vi "运行模式解析.vi"(1 "中英文选择":enum32{"中文", "English"}(radio), 2 "输入值":u8) -> (0 "输出值":string)   [LabVIEW 2013]
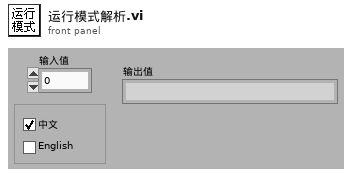
[diagram p1: front panel]
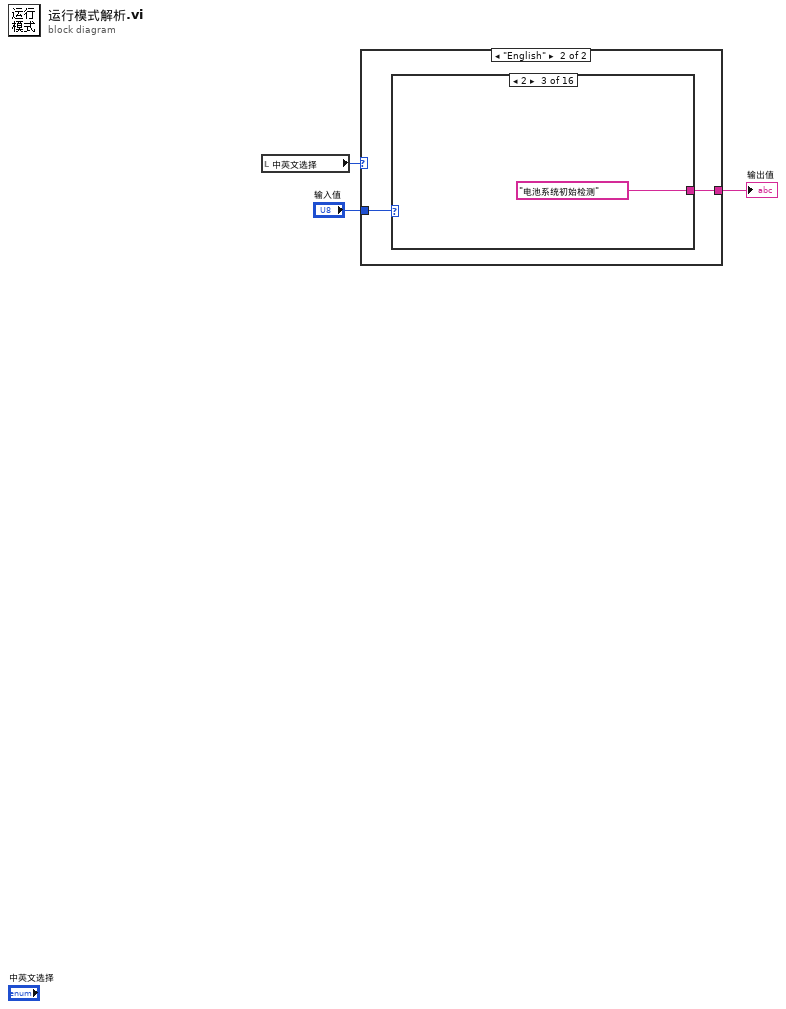
[diagram p0: block diagram]
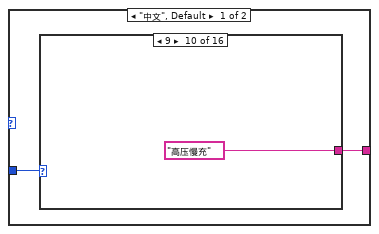
[diagram p2: hidden frame]
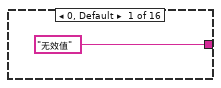
[diagram p3: hidden frame]
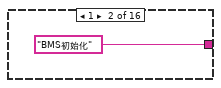
[diagram p4: hidden frame]
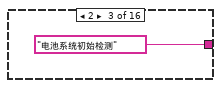
[diagram p5: hidden frame]
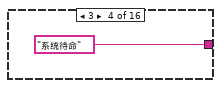
[diagram p6: hidden frame]
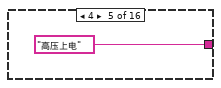
[diagram p7: hidden frame]
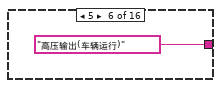
[diagram p8: hidden frame]
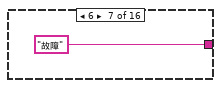
[diagram p9: hidden frame]
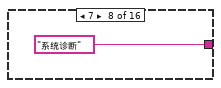
[diagram p10: hidden frame]
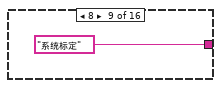
[diagram p11: hidden frame]
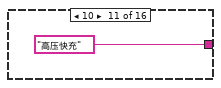
[diagram p12: hidden frame]
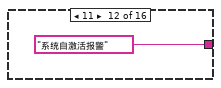
[diagram p13: hidden frame]
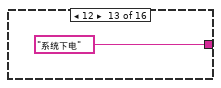
[diagram p14: hidden frame]
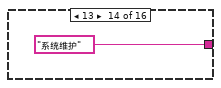
[diagram p15: hidden frame]
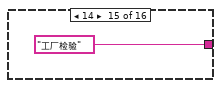
[diagram p16: hidden frame]
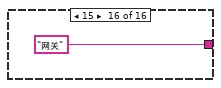
[diagram p17: hidden frame]
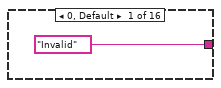
[diagram p18: hidden frame]
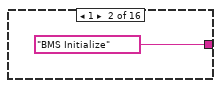
[diagram p19: hidden frame]
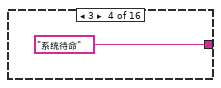
[diagram p20: hidden frame]
diagram:
  n1 = local read "中英文选择"() -> (w1:enum32{"中文", "English"})
  n2 = case shown="\"English\"" w1 {
    tunnel: "输入值" -> [w5 w23]
    tunnel: [w4 w22] -> w2
    frame "中文", Default {
      n3 = case shown="9" w5 {
        tunnel: ["无效值" "BMS初始化" "电池系统初始检测" "系统待命" "高压上电" "高压输出(车辆运行)" "故障" "系统诊断" "系统标定" "高压慢充" "高压快充" "系统自激活报警" "系统下电" "系统维护" "工厂检验" "网关"] -> w4
        frame 0, Default {
        }
        frame 1 {
        }
        frame 2 {
        }
        frame 3 {
        }
        frame 4 {
        }
        frame 5 {
        }
        frame 6 {
        }
        frame 7 {
        }
        frame 8 {
        }
        frame 9 {
        }
        frame 10 {
        }
        frame 11 {
        }
        frame 12 {
        }
        frame 13 {
        }
        frame 14 {
        }
        frame 15 {
        }
      }
    }
    frame "English" {
      n4 = case shown="2" w23 {
        tunnel: ["Invalid" "BMS Initialize" "电池系统初始检测" "系统待命" "高压上电" "高压输出(车辆运行)" "故障" "系统诊断" "系统标定" "高压慢充" "高压快充" "系统自激活报警" "系统下电" "系统维护" "工厂检验" "网关"] -> w22
        frame 0, Default {
        }
        frame 1 {
        }
        frame 2 {
        }
        frame 3 {
        }
        frame 4 {
        }
        frame 5 {
        }
        frame 6 {
        }
        frame 7 {
        }
        frame 8 {
        }
        frame 9 {
        }
        frame 10 {
        }
        frame 11 {
        }
        frame 12 {
        }
        frame 13 {
        }
        frame 14 {
        }
        frame 15 {
        }
      }
    }
  }
  "输出值" <- w2
